vi "Read from OPC Server.vi"() -> ()   [LabVIEW 2017]
panel:
  in  "Stop Button":bool
  out "Numeric Control":dbl=22.0
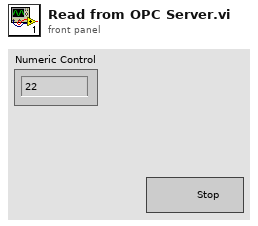
[diagram p1: front panel]
types:
  T1 = enum16{"Read", "Write", "ReadWrite", "BufferedRead", "BufferedReadWrite"}
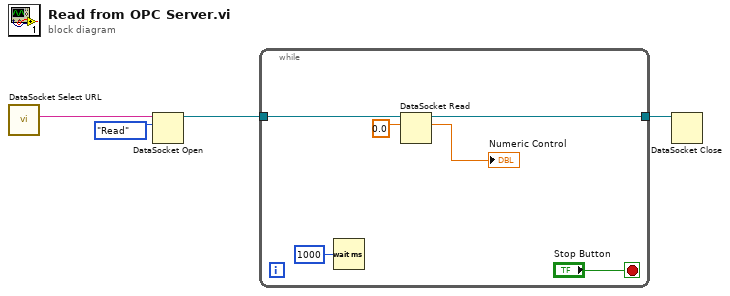
[diagram p0: block diagram]
diagram:
  n1 = call <vilib>:"DataSocket Select URL.vi"() -> ("URL"=w1:string)  [unwired: 9 in, 2 out]
  n2 = DataSocket Open(10:T1."Read" ("mode"), 11:w1) -> (3:w4:refnum<k13>)  [unwired: 2 in, 1 out]
  n3 = while {
    tunnel: w4 -> [w8]
    tunnel: [w7] -> w3
    stop <- "Stop Button" stop-if-true
    n4 = Wait (ms)(milliseconds to wait=u32 1000) -> ()  [unwired: 1 out]
    n5 = DataSocket Read(10:0.0 ("Numeric Control"), 11:w8) -> (2:→"Numeric Control":dbl, 3:w7:refnum<k13>)  [unwired: 3 in, 5 out]
  }
  n6 = DataSocket Close(11:w3) -> ()  [unwired: 2 in, 2 out]
